vi "Get Variables.vi"(8 "error in (no error)":errorcluster, 11 "Message Popup in":refnum<class "SMU.lvclass">) -> (0 "error out":errorcluster, 2 "Variables":variant, 3 "Message Popup out":refnum<class "SMU.lvclass">)   [LabVIEW 2016, in "SMU.lvclass"]
uses:
  SMU.lvclass
  SMU.lvclass/SMU.ctl
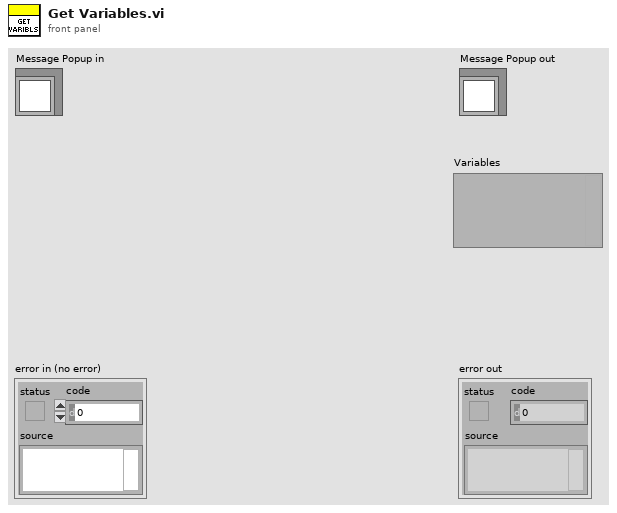
[diagram p1: front panel]
types:
  T1 = typedef "SMU.lvclass/Variables.ctl" = cluster{"instaddress":variant, "instname":string, "channel":string, "volt":dbl, "icurrent":dbl}
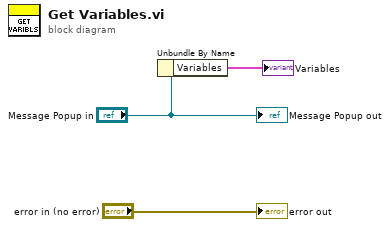
[diagram p0: block diagram]
diagram:
  n1 = Unbundle By Name("Message Popup in") -> ("Variables"=→"Variables":T1)
  "error out" <- "error in (no error)"
  "Message Popup out" <- "Message Popup in"
